vi "Main.vi"() -> ()   [LabVIEW 2019]
panel:
  out "LED":bool
  out "Signals":string
  in  "Signals":path
  in  "Java Directory":path=path ""
  in  "JAVA":bool
  in  "SIDES":bool
  out "CHANGES":dbl
  out "rest":dbl[](array[numeric])
  out "peak -":dbl[](array[numeric])
  out "peak +":dbl[](array[numeric])
  out "Release":bool
  out "Release eye controller  when LED turns RED":bool
  out "Horizontal EOG":dbl[](graph)
  out "Vertical EOG":dbl[](graph)
  in  "STOP":bool
  in  "DOWN":bool
  in  "UP":bool
  in  "L":bool
  in  "R":bool
  # "MOVEMENT SIMULATION"
  # "HORIZONTAL"
  # "VERTICAL"
  # "FRONTAL"
  # "Release eye controller  when LED turns RED"
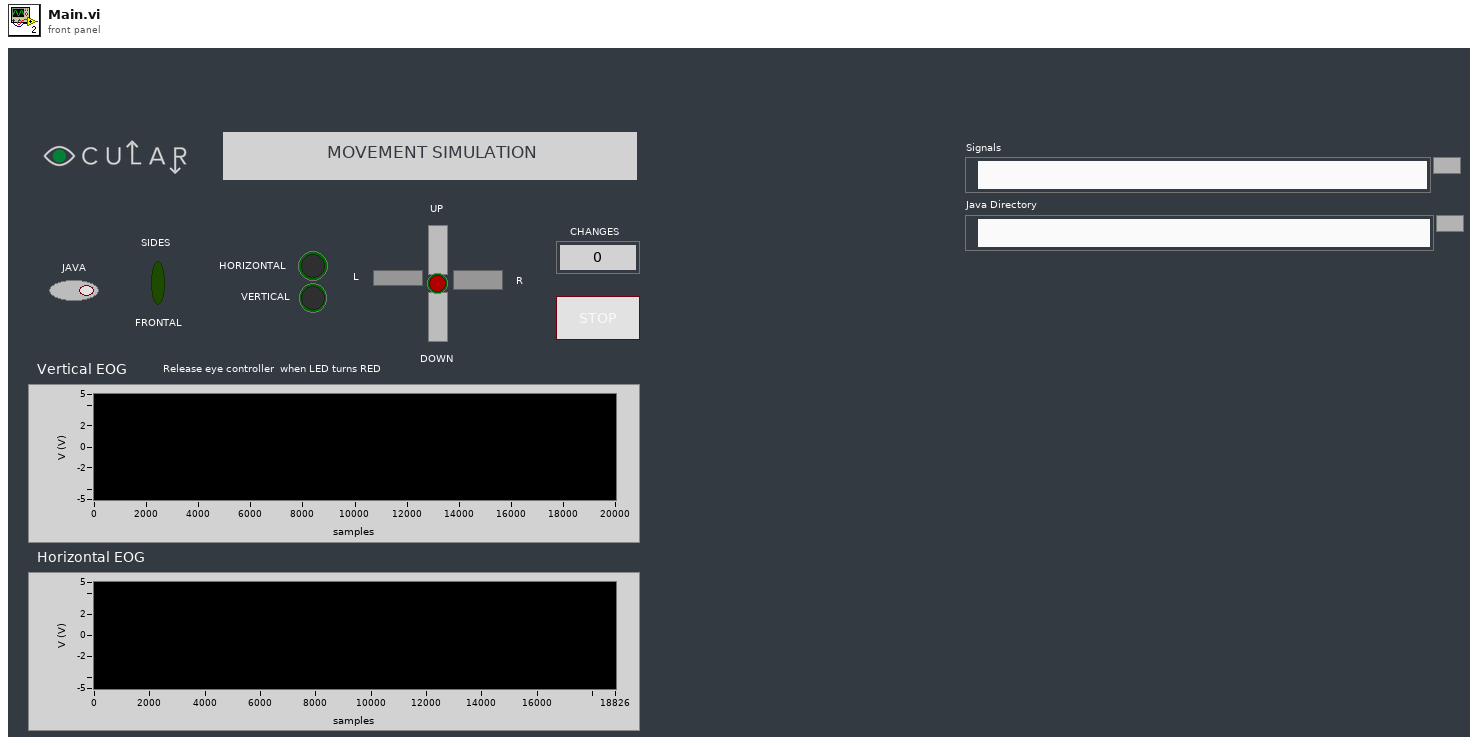
[diagram p1: front panel]
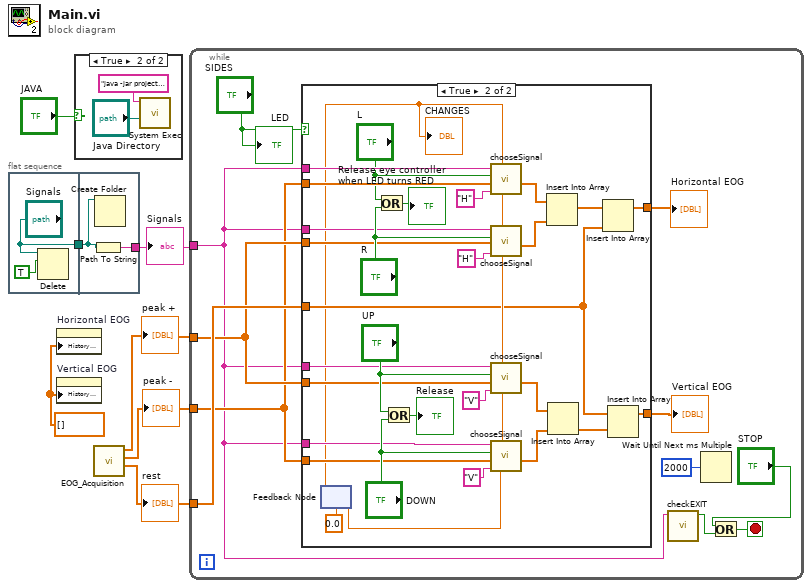
[diagram p0: block diagram]
diagram:
  w1 = dbl[] [] ("History Data")
  n1 = flat-sequence {
    tunnel: ["Signals"] -> w6
    tunnel: w6 -> [w10]
    tunnel: [w11] -> w2
    frame #0 {
      n2 = Delete(path (use dialog)="Signals", entire hierarchy (F)=TRUE) -> ()  [unwired: 3 in, 3 out]
    }
    frame #1 {
      n3 = Path To String(path=w10) -> (string=w11:string)
      n4 = Create Folder(path (use dialog)=w10) -> ()  [unwired: 2 in, 3 out]
    }
  }
  n5 = property on="Horizontal EOG" class="WFChart (strict)"("History Data"=w1) -> ()  [unwired: 2 in, 2 out]
  n6 = property on="Vertical EOG" class="WFChart (strict)"("History Data"=w1) -> ()  [unwired: 2 in, 2 out]
  n7 = case shown="True" "JAVA" {
    frame False {
    }
    frame True {
      n8 = call <vilib>:"System Exec.vi"("working directory"="Java Directory", "command line"="java -jar project.jar") -> ()  [unwired: 6 in, 4 out]
    }
  }
  n9 = call "EOG_Acquisition.vi"() -> ("Rest"=w3:dbl[], "Negative"=w4:dbl[], "Positive"=w5:dbl[])  [unwired: 8 in, 1 out]
  "peak +" <- w5
  "peak -" <- w4
  "rest" <- w3
  n10 = while {
    tunnel: w2 -> [w14]
    tunnel: w5 -> [w20]
    tunnel: w4 -> [w19]
    tunnel: w3 -> [w21]
    stop <- w17 stop-if-true
    n11 = case shown="True" "SIDES" {
      tunnel: [w25 w54] -> w24
      tunnel: [w25 w52] -> w22
      tunnel: w14 -> [_ w37]
      tunnel: w19 -> [_ w47]
      tunnel: w20 -> [_ w45]
      tunnel: w20 -> [_ w40]
      tunnel: w19 -> [_ w36]
      tunnel: w21 -> [w25 w35]
      tunnel: w14 -> [_ w30]
      tunnel: w14 -> [_ w29]
      tunnel: w14 -> [_ w28]
      frame False {
      }
      frame True {
        n12 = feedback #1(0.0) -> (w26:dbl)
        "CHANGES" <- w26
        n13 = Or(x="L", y="R") -> (x .or. y?=→"Release eye controller  when LED turns RED":bool)
        n14 = Or(x="UP", y="DOWN") -> (x .or. y?=→"Release":bool)
        n15 = call "chooseSignal.vi"("countIN"=w26, "Direction"="H", "signalIN"=w47, "chosen?"="L", "Path"=w28) -> ("signalOUT"=w51:dbl[], "countOUT"=w50:dbl)  [unwired: 5 in]
        n16 = call "chooseSignal.vi"("countIN"=w50, "Direction"="H", "signalIN"=w45, "chosen?"="R", "Path"=w37) -> ("signalOUT"=w48:dbl[], "countOUT"=w46:dbl)  [unwired: 5 in]
        n17 = call "chooseSignal.vi"("countIN"=w46, "Direction"="V", "signalIN"=w40, "chosen?"="UP", "Path"=w29) -> ("signalOUT"=w39:dbl[], "countOUT"=w44:dbl)  [unwired: 5 in]
        n18 = call "chooseSignal.vi"("countIN"=w44, "Direction"="V", "signalIN"=w36, "chosen?"="DOWN", "Path"=w30) -> ("signalOUT"=w38:dbl[], "countOUT"=w43:dbl)  [unwired: 5 in]
        n19 = feedback-in #1(w43) -> ()
        n20 = Insert Into Array(array=w51, new element=w48) -> (w55:dbl[])  [unwired: 1 in]
        n21 = Insert Into Array(array=w39, new element=w38) -> (w53:dbl[])  [unwired: 1 in]
        n22 = Insert Into Array(array=w55, new element=w35) -> (w54:dbl[])  [unwired: 1 in]
        n23 = Insert Into Array(array=w35, new element=w53) -> (w52:dbl[])  [unwired: 1 in]
      }
    }
    "Horizontal EOG" <- w24
    "Vertical EOG" <- w22
    n24 = call "checkEXIT.vi"("Path"=w14) -> ("EXIT?"=w15:bool)  [unwired: 10 in]
    n25 = Wait Until Next ms Multiple(millisecond multiple=u32 2000) -> ()  [unwired: 1 out]
    n26 = Or(x="STOP", y=w15) -> (x .or. y?=w17:bool)
    "LED" <- "SIDES"
  }
  "Signals" <- w2
